vi "blastPulse.vi"   [LabVIEW 2017]
doc: "The UDP protocol differs from TCP in that there is no error-checking with the packets of information that are sent, and thus no guarantee whatsoever that an intended recipient will actually receive a given piece of data.\n\nUDP does offer the ability to \"broadcast\" data across a network--simply specify an IP Address of all ones (255.255.255.255) to attempt to broadcast information network-wide. Keep in mind that routers and other network hardware will generally refuse to forward the broadcast beyond certain points, so the extent of the broadcast will in practice be limited."
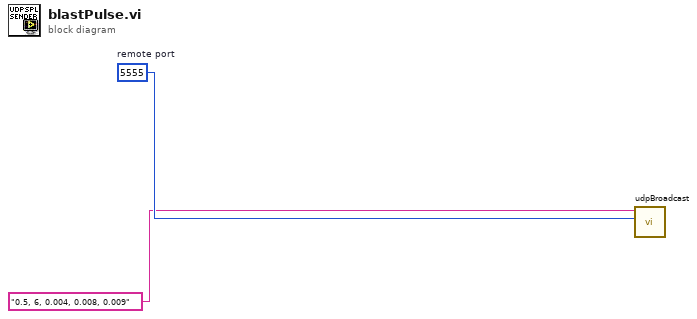
[diagram p0: block diagram]
diagram:
  w2 = u16 5555  # remote port
  n1 = call "udpBroadcast.vi"("remote port"=w2, "data in"="0.5, 6, 0.004, 0.008, 0.009") -> ()  [unwired: 10 in]
